vi "QC_Pulse_Gen.vi"() -> ()   [LabVIEW 2012]
panel:
  in  "QCpulseGen":bool
  out "QC Status":bool
  out "LOOPS":i32
  in  "stop":bool
  out "connection ID":refnum<k5>
  in  "port":u16=2101
  in  "address or name":string="QCpulseGen"
  in  "TO_Wait (mS)":i32
  out "IDN?":string
  out "error out":errorcluster
  # "QCpulseGen"
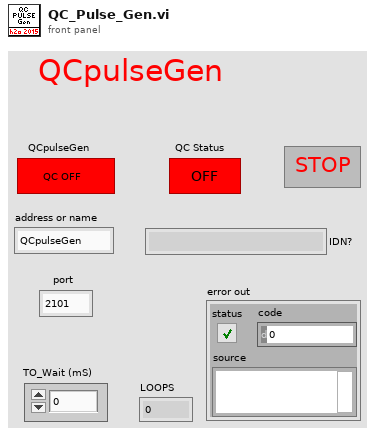
[diagram p1: front panel]
types:
  T1 = enum16{"Standard", "Buffered", "CRLF", "Immediate"}
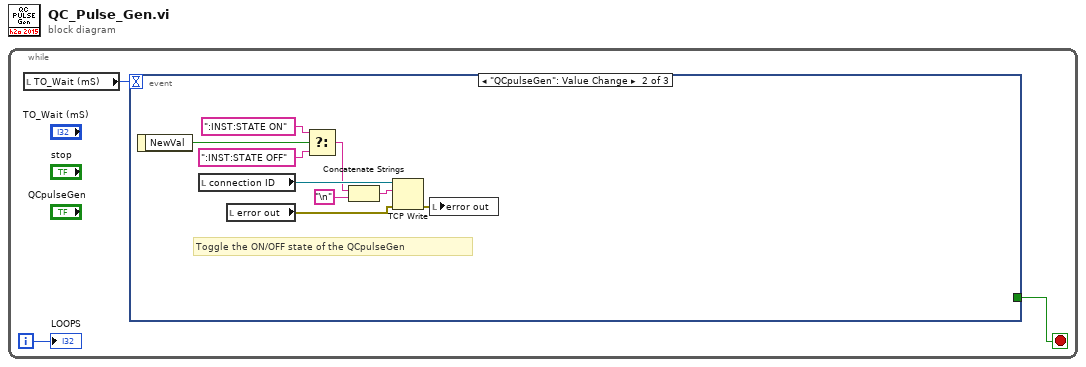
[diagram p0: block diagram]
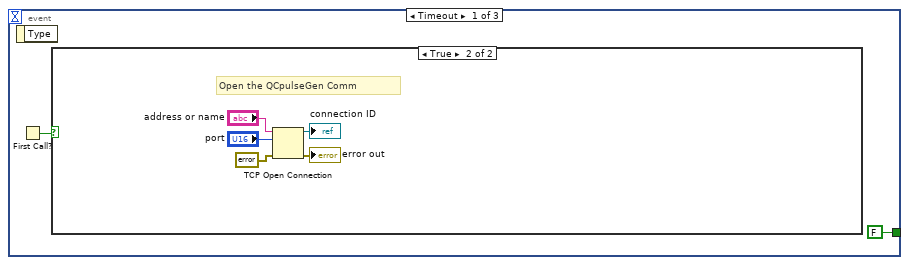
[diagram p2: hidden frame]
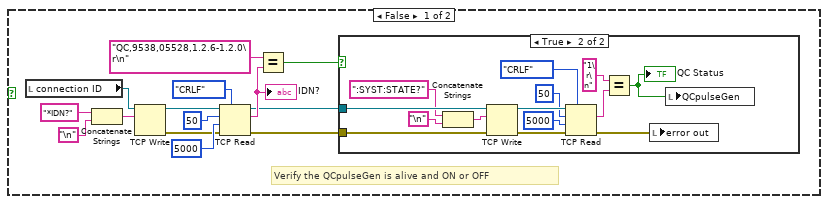
[diagram p3: hidden frame]
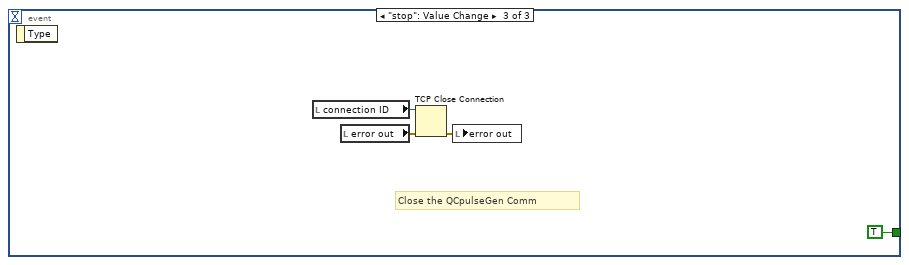
[diagram p5: hidden frame]
diagram:
  n1 = while {
    i -> [w2]
    stop <- w1 stop-if-true
    n2 = local read "TO_Wait (mS)"() -> (w3:i32)
    n3 = event shown="[1] \"QCpulseGen\": Value Change" {
      selector: _ -> [_ _ _]
      dyn-events: _ -> [_ _ _]
      timeout: w3 -> [_ _ _]
      tunnel: [FALSE _ TRUE] -> w1
      event Timeout {
        n4 = event-data() -> ()  [unwired: 1 in, 1 out]
        n5 = First Call?() -> (First Call?: T/F=w5:bool)
        n6 = case shown="True" w5 {
          frame False {
            # "Verify the QCpulseGen is alive and ON or OFF"
            n7 = local read "connection ID"() -> (w16:refnum<k5>)
            n8 = Concatenate Strings("*IDN?" ("data in"), "\n") -> (w17:string)
            n9 = TCP Write(connection ID=w16, data in=w17) -> (connection ID out=w12:refnum<k5>, error out=w11:errorcluster)  [unwired: 2 in, 1 out]
            n10 = TCP Read(connection ID=w12, bytes to read=50, error in (no error)=w11, 7:T1."CRLF" ("mode (standard)"), 9:5000 ("timeout ms (25000)")) -> (connection ID out=w7:refnum<k5>, data out=w9:string, error out=w6:errorcluster)
            "IDN?" <- w9
            n11 = Equal?(x="QC,9538,05528,1.2.6-1.2.0\r\n" ("IDN? 2"), y=w9) -> (x = y?=w8:bool)
            n12 = case shown="True" w8 {
              tunnel: w7 -> [_ w33]
              tunnel: w6 -> [_ w25]
              frame False {
              }
              frame True {
                n13 = Concatenate Strings(":SYST:STATE?" ("address"), "\n") -> (w29:string)
                n14 = TCP Write(connection ID=w33, data in=w29, error in (no error)=w25) -> (connection ID out=w32:refnum<k5>, error out=w24:errorcluster)  [unwired: 1 in, 1 out]
                n15 = TCP Read(connection ID=w32, bytes to read=50, error in (no error)=w24, 7:T1."CRLF" ("mode (standard)"), 9:5000 ("timeout ms (25000)")) -> (data out=w22:string, error out=w23:errorcluster)  [unwired: 1 out]
                n16 = Equal?(x="1\r\n" ("data out"), y=w22) -> (x = y?=w20:bool)
                "QC Status" <- w20
                n17 = local write "error out"(w23) -> ()
                n18 = local write "QCpulseGen"(w20) -> ()
              }
            }
          }
          frame True {
            # "Open the QCpulseGen Comm"
            n19 = TCP Open Connection(address="address or name", remote port or service name="port", error in (no error)=errorcluster {"status"=FALSE, "code"=0, "source"=""}) -> (connection ID=→"connection ID":refnum<k5>, error out=→"error out":errorcluster)  [unwired: 2 in]
          }
        }
      }
      event "QCpulseGen": Value Change {
        # "Toggle the ON/OFF state of the QCpulseGen"
        n20 = event-data() -> ("NewVal"=w43:bool)  [unwired: 1 in]
        n21 = local read "connection ID"() -> (w45:refnum<k5>)
        n22 = local read "error out"() -> (w44:errorcluster)
        n23 = Select(t=":INST:STATE ON" ("address"), s=w43, f=":INST:STATE OFF" ("address")) -> (s? t:f=w40:string)
        n24 = Concatenate Strings(w40, "\n") -> (w46:string)
        n25 = TCP Write(connection ID=w45, data in=w46, error in (no error)=w44) -> (error out=w39:errorcluster)  [unwired: 1 in, 2 out]
        n26 = local write "error out"(w39) -> ()
      }
      event "stop": Value Change {
        # "Close the QCpulseGen Comm"
        n27 = event-data() -> ()  [unwired: 1 in, 1 out]
        n28 = local read "connection ID"() -> (w51:refnum<k5>)
        n29 = local read "error out"() -> (w50:errorcluster)
        n30 = TCP Close Connection(connection ID=w51, error in (no error)=w50) -> (error out=w49:errorcluster)  [unwired: 1 in, 1 out]
        n31 = local write "error out"(w49) -> ()
      }
    }
    "LOOPS" <- w2
  }
